vi "Configure Standard Waveform [STD] Core.vi"(4 "dc offset (0.00 V)":dbl[unit] format="%.3f", 5 "start phase (0.00 Degrees)":dbl[unit] format="%.3f", 6 "amplitude (1.00 V)":dbl[unit]=1.0 format="%.3f", 7 "frequency (1000.0 Hz)":dbl[unit]=1000.0 format="%^.2e", 8 "error in (no error)":errorcluster, 9 "waveform (Sine)":i32(ring)=1 items=["Sine"=1, "Square"=2, "Triangle"=3, "Ramp Up"=4, "Ramp Down"=5, "DC"=6], 10 "channel name (\"CHANNEL1\")":string="CHANNEL1", 11 "CS++Fgen in":refnum<class "CS++Fgen.lvclass">) -> (0 "error out":errorcluster, 3 "CS++Fgen out":refnum<class "CS++Fgen.lvclass">)   [LabVIEW 2013, in "CS++Fgen.lvlib" / "CS++Fgen.lvclass"]
doc: "This VI configures the properties of the function generator that affect standard waveform generation. These properties are the waveform, amplitude, DC offset, frequency, and start phase.\n\nNotes:\n\n(1) This VI is part of the IviFgenStdFunc [STD] extension group."
uses:
  CS++Fgen.lvclass
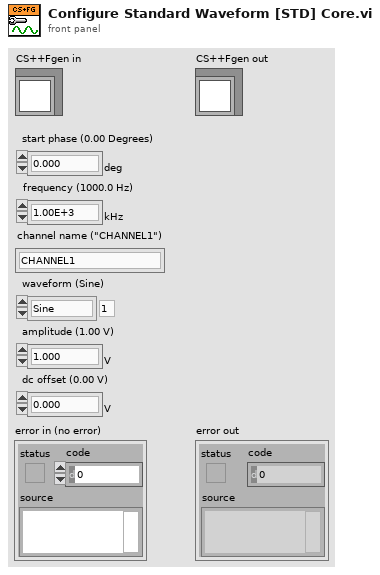
[diagram p1: front panel]
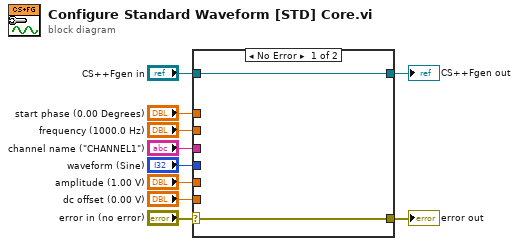
[diagram p0: block diagram]
diagram:
  n1 = case shown="No Error" "error in (no error)" {
    selector: "error in (no error)" -> [w11 w14]
    tunnel: [w11 w14] -> w9
    tunnel: [w12 w13] -> w7
    tunnel: "CS++Fgen in" -> [w12 w13]
    tunnel: "channel name (\"CHANNEL1\")" -> [_ _]
    tunnel: "start phase (0.00 Degrees)" -> [_ _]
    tunnel: "frequency (1000.0 Hz)" -> [_ _]
    tunnel: "dc offset (0.00 V)" -> [_ _]
    tunnel: "waveform (Sine)" -> [_ _]
    tunnel: "amplitude (1.00 V)" -> [_ _]
    frame No Error {
    }
    frame Error {
    }
  }
  "error out" <- w9
  "CS++Fgen out" <- w7
